vi "onStart.vi"(8 "error in (no error)":errorcluster, 11 "Client in":refnum<class "Client.lvclass">) -> (0 "error out":errorcluster, 3 "Client out":refnum<class "Client.lvclass">)   [LabVIEW 2013, in "MQTT Client.lvlib" / "Client.lvclass"]
uses:
  Client.lvclass
  Client.lvclass/Client.ctl
  Session.Client/Session.Client.lvclass
  <vilib>/LabVIEW Open Source Project/MQTT Connection/MQTT_Base/Base Class/MQTT_Base.lvclass
  <vilib>/LabVIEW Open Source Project/MQTT Connection/MQTT_Base/Session/Session.lvclass
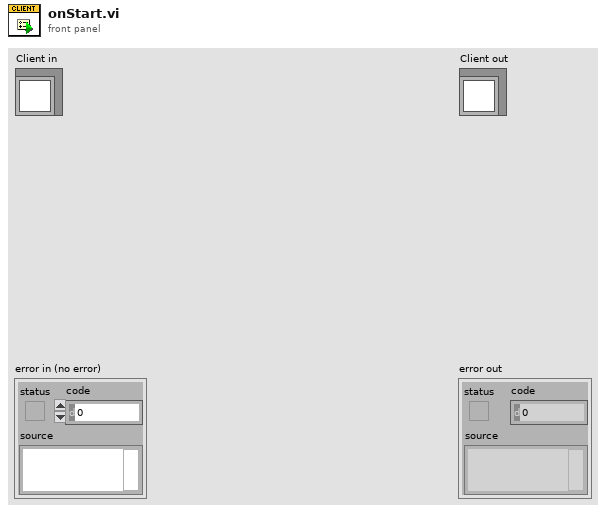
[diagram p1: front panel]
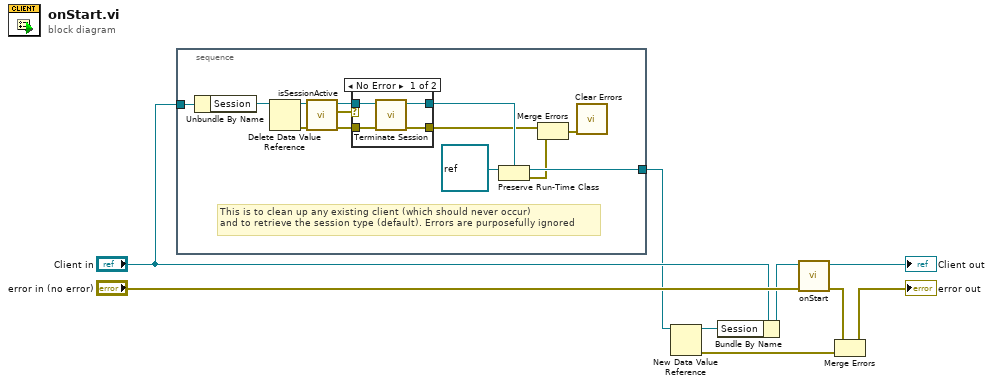
[diagram p0: block diagram]
diagram:
  n1 = stacked-sequence {
    tunnel: "Client in" -> [w21]
    tunnel: [w13] -> w1
    frame #0 {
      # "This is to clean up any existing client (which should never occur)\nand to retrieve the session type (default). Errors are purposefully ignored"
      n2 = Unbundle By Name(w21) -> ("Session"=w20:refnum<data-value>)
      n3 = Delete Data Value Reference(data value reference=w20) -> (data value=w18:refnum<class "Session.Client.lvclass">, error out=w16:errorcluster)  [unwired: 1 in]
      n4 = call <vilib>:"isSessionActive.vi"("Session in"=w18) -> ("error out"=w17:errorcluster, "Session out"=w19:refnum<class "Session.Client.lvclass">)  [unwired: 9 in]
      n5 = case shown="No Error" w17 {
        tunnel: [w25 w27] -> w12
        tunnel: w19 -> [w24 w26]
        tunnel: w16 -> [w23 w27]
        tunnel: [w22 w26] -> w15
        frame No Error {
          n6 = call <vilib>:"Terminate Session.vi"("error in (no error)"=w23, "Session in"=w24) -> ("error out"=w25:errorcluster, "Session out"=w22:refnum<class "Session.Client.lvclass">)  [unwired: 7 in, 1 out]
        }
        frame Error {
        }
      }
      n7 = Preserve Run-Time Class(object in=refnum<class> refnum ("LabVIEW Object"), 2:w15) -> (object out=w13:refnum<class "Session.Client.lvclass">, error out=w11:errorcluster)  [unwired: 1 in]
      n8 = Merge Errors(w12, w11) -> (w10:errorcluster)
      n9 = call <vilib>:"Clear Errors.vi"("error in (no error)"=w10) -> ()  [unwired: 6 in, 1 out]
    }
  }
  n10 = New Data Value Reference(data value=w1) -> (data value reference=w7:refnum<data-value>, error out=w6:errorcluster)  [unwired: 1 in]
  n11 = Bundle By Name(cluster="Client in", "Session"=w7) -> (w3:refnum<class "Client.lvclass">)
  n12 = call-parent "onStart.vi"("error in (no error)"="error in (no error)", "MQTT_Base in"=w3) -> ("error out"=w5:errorcluster, "MQTT_Base out"=→"Client out":refnum<class "Client.lvclass">)  [unwired: 8 in]
  n13 = Merge Errors(w5, w6) -> (→"error out":errorcluster)
